vi "Request current CH1(SubVI).vi"() -> (3 "Request current CH1 / X":string)   [LabVIEW 2018]
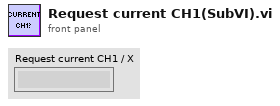
[diagram p1: front panel]
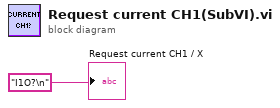
[diagram p0: block diagram]
diagram:
  "Request current CH1 / X" <- "I1O?\n" ("format string")
